vi "MC5e Sqauds in Unit Strings.vi"(8 "error in":errorcluster, 11 "Unit index":i32) -> (0 "error out":errorcluster, 3 "Squad Strings":string[](array[string]))   [LabVIEW 2020]
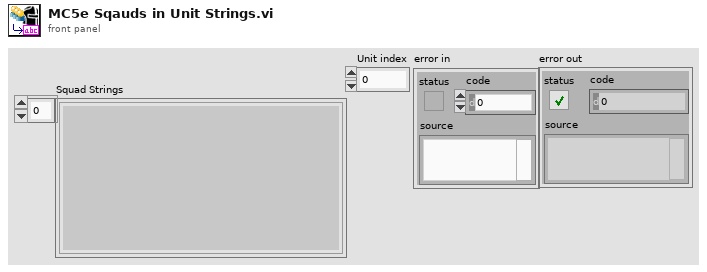
[diagram p1: front panel]
types:
  T1 = typedef "MC5e Unit.ctl" = cluster{"Unit Fatigue Level":enum16{"Not Fatigued", "Fatigued", "Seriously Fatigued"}, "Flying Unit":bool, "Mounted Unit":bool, "Defending from Stronghold":bool, "Difficult Terrain Types":T2, "Squads in Unit":T3[], "Unit Info":T5, "Range":i32, "BR":i32, "Speed":i32, "Morale":i32, "Current BR":i32, "Location":T6, "Capacity %":i32}
  T2 = typedef "MC5e Terrain types.ctl" = i32[]
  T3 = typedef "MC5e Squad_Info.ctl" = cluster{"Squad Name":string, "# Soldiers":u16, "Battle Rating":u16, "Flying":bool, "Mounted":bool, "Speed":u16, "Range":u16, "Morale":i32, "Max Endurance":u16, "Current Endurance":i32, "Size":T4, "Space Taken":u16, "Difficult Terrain":i32[], "CR":u16, "Special / Notes":string}
  T4 = typedef "MC5e Size_Categories.ctl" = enum16{"Tiny", "Small", "Medium", "Large", "Huge", "Gargantuan"}
  T5 = typedef "MC5e Unit Header.ctl" = cluster{"Unit Name":string, "Unit Commander":string, "Morale Mod":i32, "BR Mod":i32, "Defense Mod":i32, "Speed Mod":i32, "Unit Notes":string, "Attack Mod":i32, "Unit Wins+ Losses-":i32, "Commander Charisma Bonus":i32}
  T6 = typedef "Location.ctl" = cluster{"X coordinate":dbl, "Y coordinate":dbl}
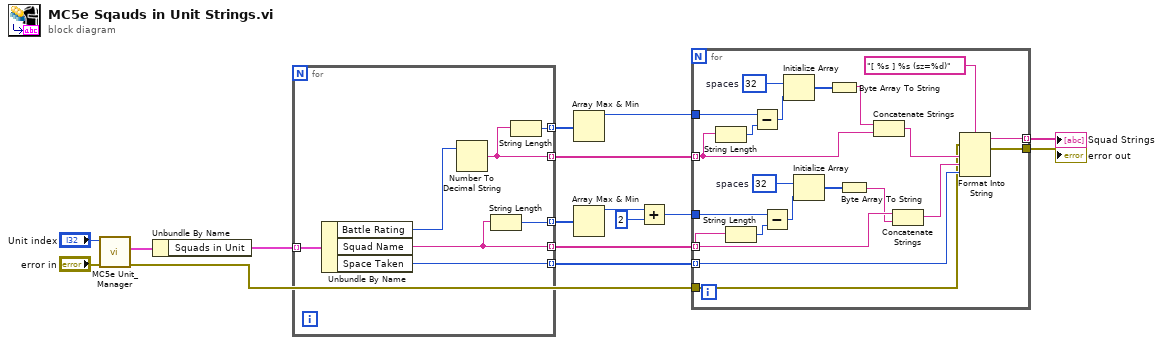
[diagram p0: block diagram]
diagram:
  n1 = call "MC5e Unit_Manager.vi"("error in"="error in", "index (get/delete)"="Unit index") -> ("error out"=w2:errorcluster, "Unit"=w5:T1)  [unwired: 6 in, 2 out]
  n2 = Unbundle By Name(w5) -> ("Squads in Unit"=w4:T3[])
  n3 = for {
    tunnel: [w19] -> w13 mode=indexing
    tunnel: [w23] -> w16 mode=indexing
    tunnel: [w18] -> w11 mode=indexing
    tunnel: [w22] -> w12 mode=indexing
    tunnel: [w21] -> w7 mode=indexing
    tunnel: w4 -> [w17] mode=indexing
    n4 = Unbundle By Name(w17) -> ("Battle Rating"=w20:u16, "Squad Name"=w19:string, "Space Taken"=w18:u16)
    n5 = Number To Decimal String(number=w20) -> (decimal integer string=w22:string)  [unwired: 1 in]
    n6 = String Length(string=w19) -> (length=w23:i32)
    n7 = String Length(string=w22) -> (length=w21:i32)
  }
  n8 = Array Max & Min(array=w7) -> (max value=w8:i32)  [unwired: 3 out]
  n9 = Array Max & Min(array=w16) -> (max value=w15:i32)  [unwired: 3 out]
  n10 = Add(x=w15, y=2) -> (x+y=w9:i32)
  n11 = for {
    tunnel: w13 -> [w36] mode=indexing
    tunnel: w12 -> [w28] mode=indexing
    tunnel: w11 -> [w43] mode=indexing
    tunnel: [w42] -> w10 mode=indexing
    tunnel: w9 -> [w40]
    tunnel: w8 -> [w29]
    tunnel: w2 -> [w25]
    tunnel: [w24] -> w1
    w32 = u8 32  # spaces
    w38 = u8 32  # spaces
    n12 = String Length(string=w28) -> (length=w30:i32)
    n13 = String Length(string=w36) -> (length=w41:i32)
    n14 = Subtract(x=w29, y=w30) -> (x-y=w33:i32)
    n15 = Subtract(x=w40, y=w41) -> (x-y=w37:i32)
    n16 = Initialize Array(w32, w33) -> (w31:u8[])
    n17 = Initialize Array(w38, w37) -> (w39:u8[])
    n18 = Byte Array To String(unsigned byte array=w31) -> (string=w27:string)
    n19 = Byte Array To String(unsigned byte array=w39) -> (string=w35:string)
    n20 = Concatenate Strings(w27, w28) -> (w26:string)
    n21 = Concatenate Strings(w36, w35) -> (w34:string)
    n22 = Format Into String(format string="[ %s ] %s (sz=%d)", error in=w25, w26, w34, w43) -> (resulting string=w42:string, error out=w24:errorcluster)  [unwired: 1 in]
  }
  "Squad Strings" <- w10
  "error out" <- w1
